vi "Frontend FPP v2.0.vi"() -> ()   [LabVIEW 2016]
panel:
  in  "Gate 2":T1={"Gate Start"=0.0, "Gate Stop"=2.0, "Gate Step (linear only)"=1.0, "Gate Compliance"=0.0001, "Gate PComp"=0.0, "Range mode"=0, "Range"=6} {"Range" max=11 scale=0.0..11.0; "Range mode" items=["Auto", "Limited", "Fixed"]; "Gate PComp" format="%^.2e"; "Gate Compliance" format="%^.2e"; "Gate Step (linear only)" format="%^.4e"; "Gate Stop" format="%^.4e"; "Gate Start" format="%^.4e"}
  in  "Drain":T2={"Drain Start"=0.0, "Drain Stop"=2.0, "Drain Compliance"=0.0001, "Drain Step"=1.0, "Drain PComp"=0.0, "Range mode"=0, "Range"=6} {"Range" max=11 scale=0.0..11.0; "Range mode" items=["Auto", "Limited", "Fixed"]; "Drain PComp" format="%^.2e"; "Drain Step" format="%^.4e"; "Drain Compliance" format="%^.2e"; "Drain Stop" format="%^.4e"; "Drain Start" format="%^.4e"}
  in  "Gate":T3={"Gate Start"=0.0, "Gate Stop"=2.0, "Gate Step"=1.0, "Gate Compliance"=0.0001, "Gate PComp"=0.0, "Range mode"=0, "Range"=6} {"Range" max=11 scale=0.0..11.0; "Range mode" items=["Auto", "Limited", "Fixed"]; "Gate PComp" format="%^.2e"; "Gate Compliance" format="%^.2e"; "Gate Step" format="%^.4e"; "Gate Stop" format="%^.4e"; "Gate Start" format="%^.4e"}
  in  "Drain 2":T4={"Drain Start"=0.0, "Drain Stop"=2.0, "Drain Compliance"=0.0001, "Drain Step (linear only)"=1.0, "Drain PComp"=0.0, "Range mode"=0, "Range"=6} {"Range" max=11 scale=0.0..11.0; "Range mode" items=["Auto", "Limited", "Fixed"]; "Drain PComp" format="%^.2e"; "Drain Step (linear only)" format="%^.4e"; "Drain Compliance" format="%^.2e"; "Drain Stop" format="%^.4e"; "Drain Start" format="%^.4e"}
  in  "Timings":T5={"integration time"=0, "Short/Long integration time"=0.00064, "hold time (sec)"=0.0, "delay time (sec)"=0.0, "Step Time (0 disables)"=0.0, "sweep method"=0, "Pulse period"=0.005, "Base voltage"=0.0, "Pulse width"=0.0005} {"Pulse width" min=0.0005 max=0.1 step=0.0001 format="%.4f"; "Base voltage" format="%^.4e"; "Pulse period" min=0.005 max=1.0 step=0.0001 format="%.4f"; "sweep method" items=["Continuous", "Pulsed"]; "Step Time (0 disables)" format="%.2f"; "delay time (sec)" format="%.4f"; "hold time (sec)" format="%.4f"; "Short/Long integration time" format="%^.0e"; "integration time" scale=0.0..2.0}
  in  "Panel controls":T6={"Emergency Stop"=refnum, "OutputGraph Max"=1e-05, "Text/Graph (text=false)"=FALSE} {"OutputGraph Max" format="%.2e"}
  in  "Panel Controls":T7={"Emergency Stop"=refnum, "TransGraph Max"=1e-05, "Text/Graph (text=false)"=FALSE} {"TransGraph Max" format="%.2e"}
  in  "Tab Control":enum32{"Characteristics", "Other parameters"}(tab)
  out "XY Graph 2":cluster{"Y data in":dbl[], "X data in":dbl[]}[](graph)
  in  "Integration time (long)":dbl=0.32 min=0.04 max=2.0 step=0.02 format="%.2f"
  in  "Integration time (short)":dbl=0.00064 min=8e-05 max=0.00192 step=8e-05 format="%^.0e"
  in  "Drain Range":u8(slide)=6 max=11 scale=0.0..11.0
  in  "Drain Range mode":u16(ring) items=["Auto", "Limited", "Fixed"]
  in  "Gate Range":u8(slide)=6 max=11 scale=0.0..11.0
  in  "Gate Range mode":u16(ring) items=["Auto", "Limited", "Fixed"]
  in  "Sampling mode":u32(slide) scale=0.0..4.0
  in  "Number of Samples":i32=500 min=0 step=1
  in  "Time":dbl=240.0 min=0.0 format="%.2f"
  in  "Drain":dbl=-10.0 min=-100.0 max=100.0 format="%.2f"
  in  "Gate":dbl=-60.0 min=-100.0 max=100.0 format="%.2f"
  in  "sweep method":u16(ring) items=["Continuous", "Pulsed"]
  out "Id":dbl format="%.2e"
  out "Ig":dbl format="%.2e"
  in  "Sweep Start":bool caption="Sweep start"
  in  "Interrupt run":bool
  in  "Running":bool=TRUE
  out "Path":path
  in  "integration time":u32(slide)=1 max=2 step=1 scale=0.0..2.0
  in  "sweep mode":u16(ring)=1 items=["Single", "Double"]
  in  "Transfer Start":bool
  in  "Output Start":bool
  in  "Drain: Step":dbl=-1.0 min=-100.0 max=100.0 format="%.2f"
  in  "Drain: Stop":dbl=-60.0 min=-100.0 max=100.0 format="%.2f"
  in  "Drain:Start":dbl min=-100.0 max=100.0 format="%.2f"
  in  "Gate: Step":dbl=-20.0 min=-100.0 max=100.0 format="%.2f"
  in  "Gate: Stop":dbl=-60.0 min=-100.0 max=100.0 format="%.2f"
  in  "Gate: Start":dbl min=-100.0 max=100.0 format="%.2f"
  out "XY Graph":cluster{"Y data in":dbl[], "X data in":dbl[]}[](graph)
  in  "Drain: Compliance":dbl=0.001 min=1e-12 max=0.02 format="%.8f"
  in  "Gate: Compliance":dbl=0.001 min=1e-12 max=0.02 format="%.8f"
  in  "Drain: Step":dbl=-5.0 min=-100.0 max=100.0 format="%.2f"
  in  "Drain: Stop":dbl=-10.0 min=-100.0 max=100.0 format="%.2f"
  in  "Drain:Start":dbl=-5.0 min=-100.0 max=100.0 format="%.2f"
  in  "Gate: Step":dbl=-1.0 min=-100.0 max=100.0 format="%.2f"
  in  "Gate: Stop":dbl=-60.0 min=-100.0 max=100.0 format="%.2f"
  in  "Gate: Start":dbl=10.0 min=-100.0 max=100.0 format="%.2f"
  in  "FPP - Source":u32(ring) items=["VSU1  ", "VSU2  "]
  in  "FPP - Drain":u32(ring)=1 items=["SMU1  ", "SMU2  ", "SMU3  ", "SMU4  ", "SMU5  ", "SMU6  "]
  in  "FPP - Gate":u32(ring)=2 items=["SMU1  ", "SMU2  ", "SMU3  ", "SMU4  ", "SMU5  ", "SMU6  "]
  in  "FPP - Probe 1":u32(ring) items=["SMU1  ", "SMU2  ", "SMU3  ", "SMU4  ", "SMU5  ", "SMU6  "]
  in  "FPP - Probe 2":u32(ring)=3 items=["SMU1  ", "SMU2  ", "SMU3  ", "SMU4  ", "SMU5  ", "SMU6  "]
  in  "Pulse width":dbl=0.0005 min=0.0005 max=0.1 step=0.0001 format="%.4f"
  in  "Base voltage":dbl min=-100.0 max=100.0 format="%.2f"
  in  "Pulse period":dbl=0.005 min=0.005 max=1.0 step=0.0001 format="%.4f"
  in  "Drain Power Compliance":dbl min=0.0 max=1.0 format="%.2f"
  in  "Gate Power\nCompliance":dbl min=0.0 max=1.0 format="%.2f"
  in  "OutputGraph Max":dbl=1e-05 format="%.2e"
  in  "TransGraph Max":dbl=1e-05 format="%.2e"
  in  "SPA Display":bool
  in  "Step delay /s":dbl min=0.0 max=1.0 format="%.2f"
  in  "hold time /s":dbl min=0.0 max=655.35 step=0.01 format="%.2f"
  in  "delay time /s":dbl min=0.0 max=65.535 step=0.0001 format="%.2f"
  in  "Decimal places in header":i8=1
  out "error out":errorcluster
  in  "VISA resource name in":refnum<visa-resource-name>="GPIB0::14::INSTR"
  # "Transfer Characteristics"
  # "Stress Measurements"
  # "V"
  # "V"
  # "V"
  # "Gate"
  # "V"
  # "V"
  # "V"
  # "V"
  # "Drain"
  # "V"
  # "s"
  # "Output Characteristics"
  # "V"
  # "V"
  # "V"
  # "Gate"
  # "V"
  # "V"
  # "Drain"
  # "V"
  # "For Four Point Probe measurements ONLY!"
  # "Vp1"
  # "Vp2"
  # "A"
  # "A"
  # "Pulsed mode settings"
  # "NOTE - THIS OVERRIDES THE COMPLIANCE VALUES!"
  # "A"
  # "A"
  # "Enter max power in Watts (max 1W)"
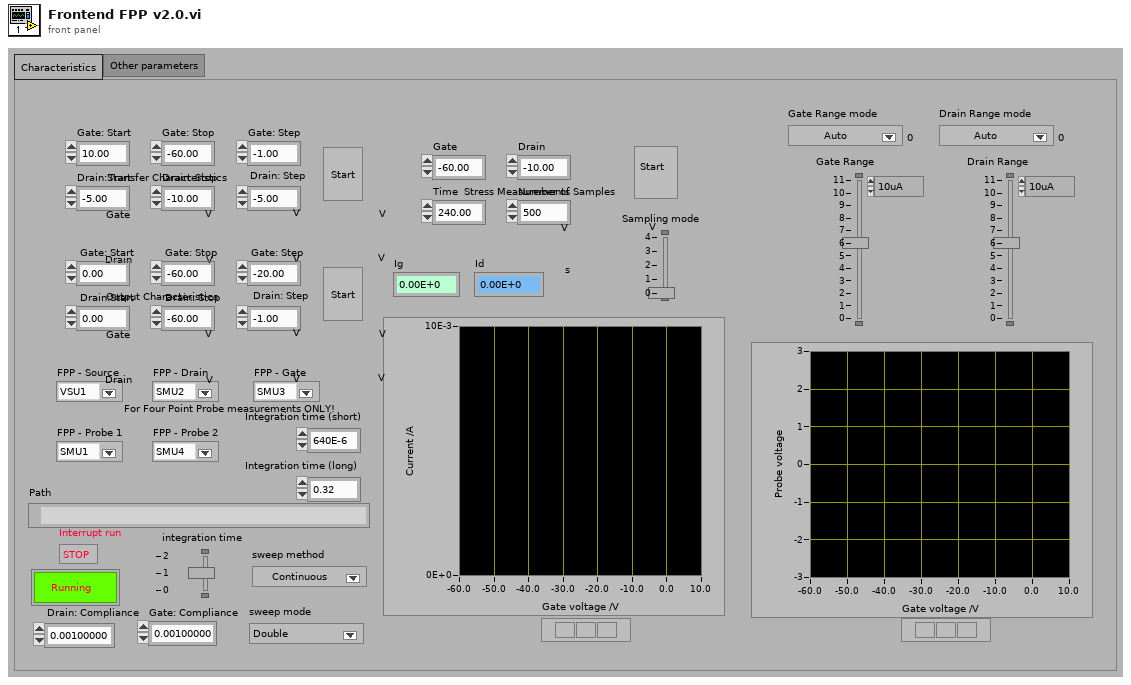
[diagram p1: front panel]
types:
  T1 = cluster{"Gate Start":dbl, "Gate Stop":dbl, "Gate Step (linear only)":dbl, "Gate Compliance":dbl, "Gate PComp":dbl, "Range mode":u16, "Range":u8}
  T2 = cluster{"Drain Start":dbl, "Drain Stop":dbl, "Drain Compliance":dbl, "Drain Step":dbl, "Drain PComp":dbl, "Range mode":u16, "Range":u8}
  T3 = cluster{"Gate Start":dbl, "Gate Stop":dbl, "Gate Step":dbl, "Gate Compliance":dbl, "Gate PComp":dbl, "Range mode":u16, "Range":u8}
  T4 = cluster{"Drain Start":dbl, "Drain Stop":dbl, "Drain Compliance":dbl, "Drain Step (linear only)":dbl, "Drain PComp":dbl, "Range mode":u16, "Range":u8}
  T5 = cluster{"integration time":u32, "Short/Long integration time":dbl, "hold time (sec)":dbl, "delay time (sec)":dbl, "Step Time (0 disables)":dbl, "sweep method":u16, "Pulse period":dbl, "Base voltage":dbl, "Pulse width":dbl}
  T6 = cluster{"Emergency Stop":refnum<vi>, "OutputGraph Max":dbl, "Text/Graph (text=false)":bool}
  T7 = cluster{"Emergency Stop":refnum<vi>, "TransGraph Max":dbl, "Text/Graph (text=false)":bool}
  T8 = cluster{"V2 Start":dbl, "V2 Step":dbl, "Number of points":i32}
  T9 = enum16{"open", "replace", "create", "open or create", "replace or create", "replace or create with confirmation"}
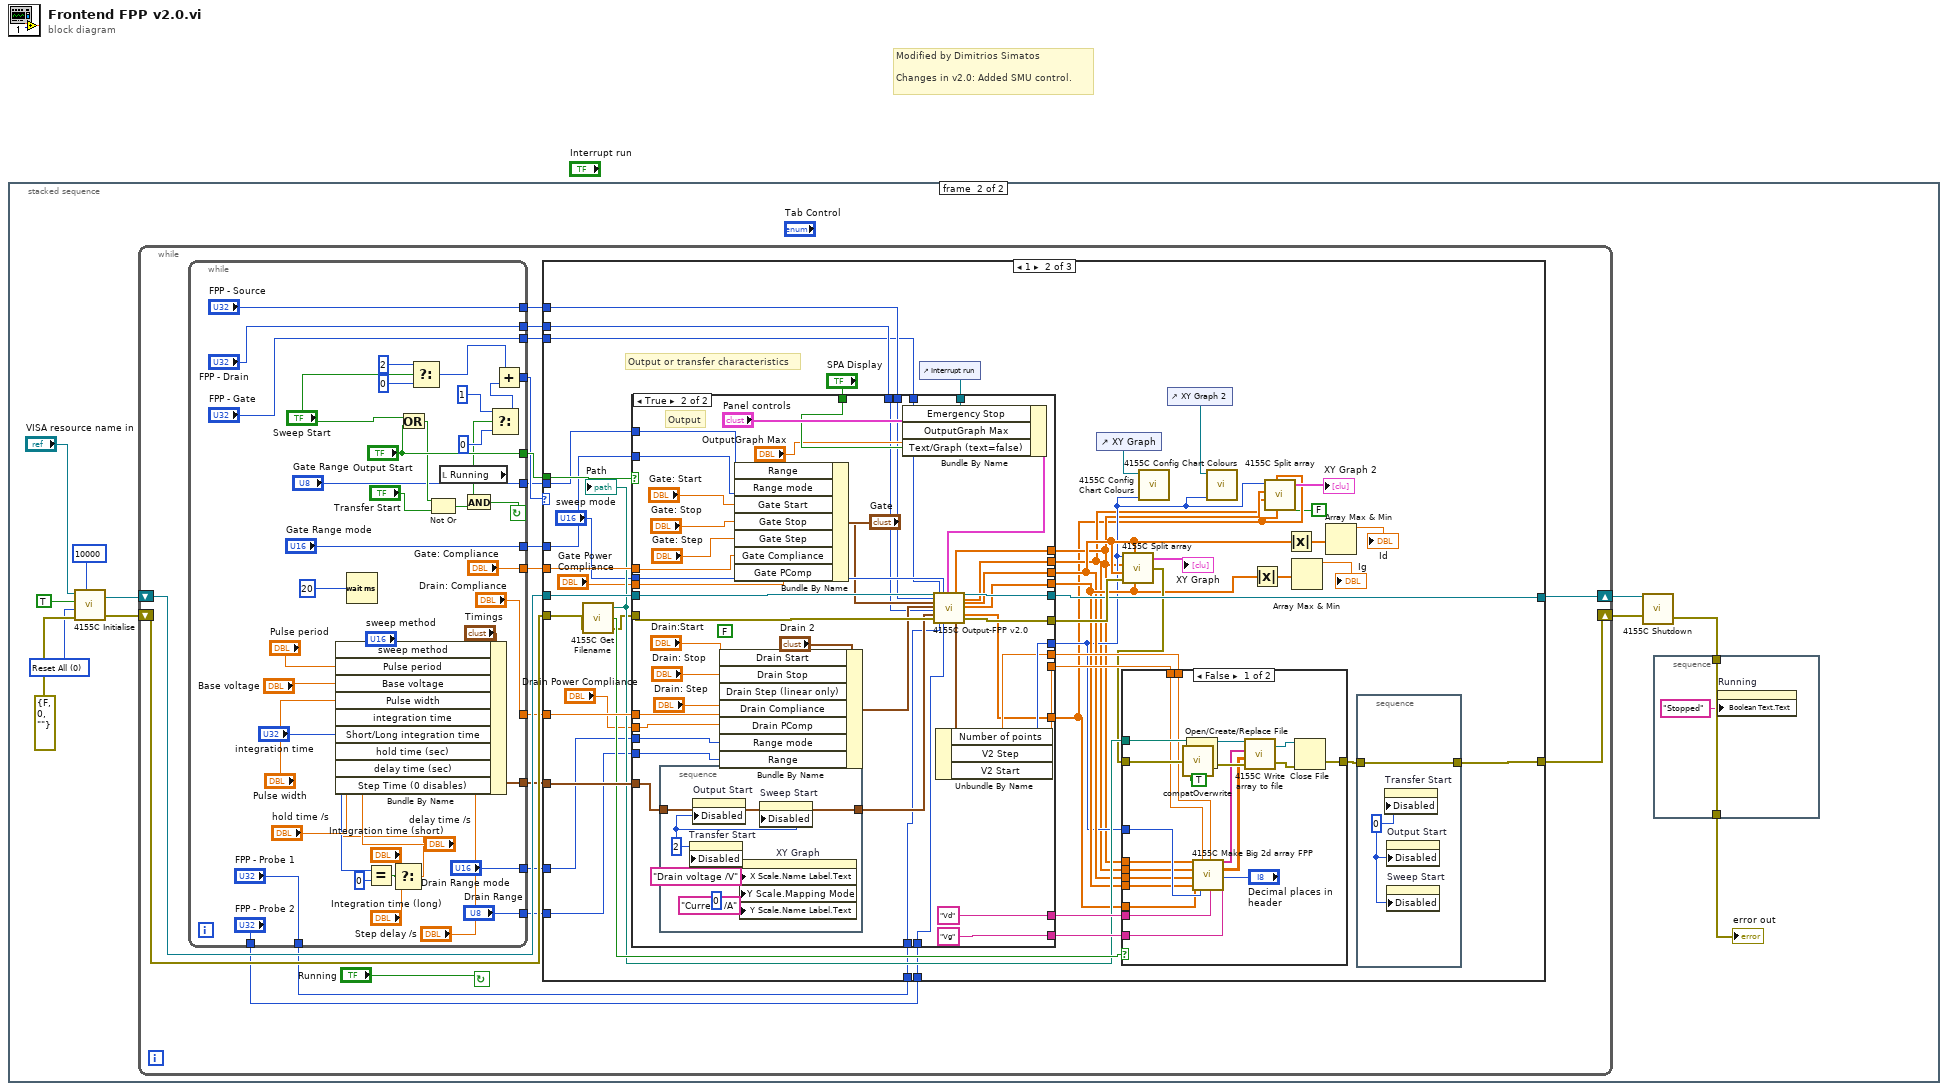
[diagram p0: block diagram]
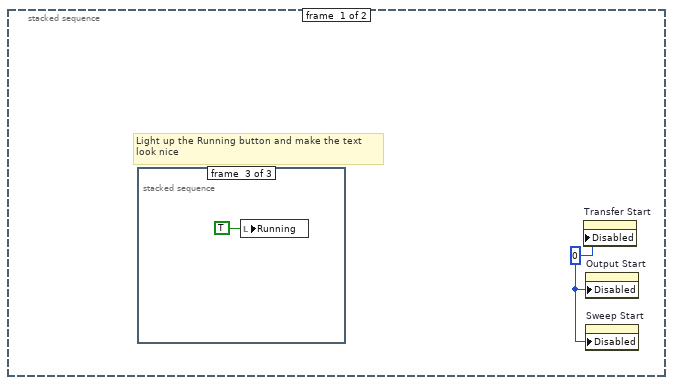
[diagram p2: hidden frame]
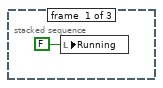
[diagram p3: hidden frame]
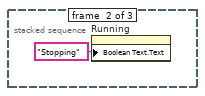
[diagram p4: hidden frame]
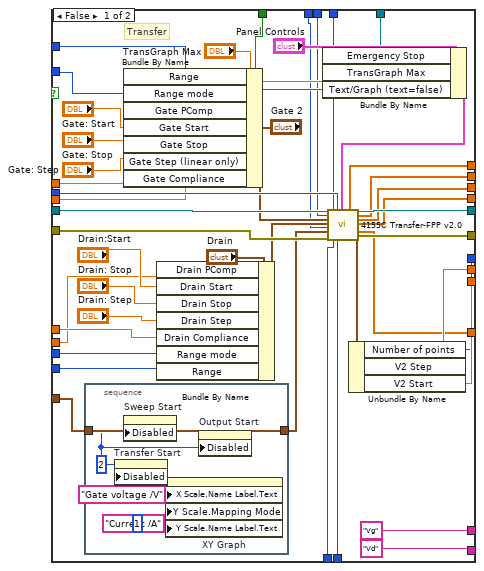
[diagram p7: hidden frame]
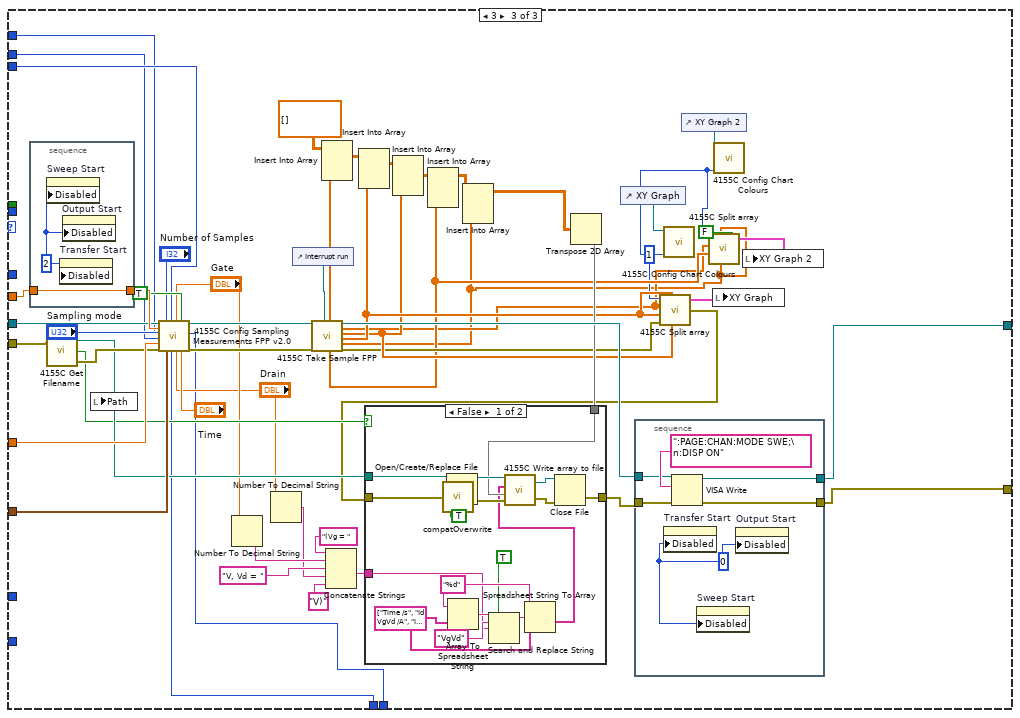
[diagram p8: hidden frame]
diagram:
  # "Modified by Dimitrios Simatos\n\nChanges in v2.0: Added SMU control."
  n1 = stacked-sequence {
    frame #0 {
      w1 = u8 0 ("Disabled")
      # "Light up the Running button and make the text\nlook nice"
      n2 = stacked-sequence {
        frame #0 {
          n3 = local write "Running"(FALSE ("Running")) -> ()
        }
        frame #1 {
          n4 = property on="Running" class="Bool (strict)"("Boolean Text.Text"="Stopping") -> ()  [unwired: 2 in, 2 out]
        }
        frame #2 {
          (unwired) FALSE ("Running")
          n5 = local write "Running"(TRUE ("Running")) -> ()
        }
      }
      n6 = property on="Transfer Start" class="Bool (strict)"("Disabled"=w1) -> ()  [unwired: 2 in, 2 out]
      n7 = property on="Output Start" class="Bool (strict)"("Disabled"=w1) -> ()  [unwired: 2 in, 2 out]
      n8 = property on="Sweep Start" class="Bool (strict)"("Disabled"=w1) -> ()  [unwired: 2 in, 2 out]
    }
    frame #1 {
      w11 = u16 0 items=["Reset All", "Partial reset"] ("Type of reset")
      n9 = call "4155C Initialise.vi"("VISA resource name in"="VISA resource name in", "Reset"=TRUE, "Type of reset"=w11, "error in (no error)"=errorcluster {"status"=FALSE, "code"=0, "source"=""}, "VISA Timeout Value"=u32 10000) -> ("VISA Resource Name out"=w10:refnum<visa-resource-name>, "error out"=w9:errorcluster)
      n10 = while {
        shift-left: w10 -> [w29]
        shift-right: [w31] -> w5
        shift-left: w9 -> [w30]
        shift-right: [w32] -> w6
        stop <- "Running" continue-if-true
        n11 = while {
          tunnel: ["Gate Range"] -> w21
          tunnel: ["Gate Range mode"] -> w22
          tunnel: ["Drain Range"] -> w23
          tunnel: ["Drain Range mode"] -> w24
          tunnel: ["Drain: Compliance"] -> w25
          tunnel: [w59] -> w26
          tunnel: ["Gate: Compliance"] -> w27
          tunnel: [w65] -> w28
          tunnel: ["Output Start"] -> w33
          tunnel: ["FPP - Source"] -> w20
          tunnel: ["FPP - Drain"] -> w19
          tunnel: ["FPP - Gate"] -> w18
          tunnel: ["FPP - Probe 2"] -> w17
          tunnel: ["FPP - Probe 1"] -> w16
          stop <- w74 continue-if-true
          n12 = Wait (ms)(milliseconds to wait=u32 20) -> ()  [unwired: 1 out]
          n13 = Equal?(x="integration time", y=u32 0) -> (x = y?=w56:bool)
          n14 = Select(t="Integration time (short)", s=w56, f="Integration time (long)") -> (s? t:f=w53:dbl)
          n15 = Bundle By Name(cluster="Timings", "sweep method"="sweep method", "Pulse period"="Pulse period", "Base voltage"="Base voltage", "Pulse width"="Pulse width", "integration time"="integration time", "Short/Long integration time"=w53, "hold time (sec)"="hold time /s", "delay time (sec)"="delay time /s", "Step Time (0 disables)"="Step delay /s") -> (w59:T5)
          n16 = Or(x="Sweep Start", y="Output Start") -> (x .or. y?=w71:bool)
          n17 = Select(t=i8 2, s="Sweep Start", f=i8 0) -> (s? t:f=w41:i8)
          n18 = Not Or(1:"Transfer Start", 2:w71) -> (0:w73:bool)
          n19 = local read "Running"() -> (w68:bool)
          n20 = And(x=w68, y=w73) -> (x .and. y?=w74:bool)
          n21 = Select(t=i8 1, s=w68, f=i8 0) -> (s? t:f=w64:i8)
          n22 = Add(x=w41, y=w64) -> (x+y=w65:i8)
        }
        n23 = case shown="1" w28 {
          tunnel: w33 -> [_ w124 _]
          tunnel: w26 -> [_ w123 w296]
          tunnel: w27 -> [_ w122 w304]
          tunnel: w25 -> [_ w121 w300]
          tunnel: [w77 w112 w302] -> w32
          tunnel: [w76 w115 w303] -> w31
          tunnel: w30 -> [w77 w106 w291]
          tunnel: w29 -> [w76 w114 w290]
          tunnel: w24 -> [_ w96 _]
          tunnel: w23 -> [_ w95 _]
          tunnel: w22 -> [_ w94 _]
          tunnel: w21 -> [_ w93 _]
          tunnel: w20 -> [_ w82 w255]
          tunnel: w19 -> [_ w81 w254]
          tunnel: w18 -> [_ w80 w256]
          tunnel: w17 -> [_ w79 w253]
          tunnel: w16 -> [_ w78 w252]
          frame 0, Default {
            # "Someone's deselected the running button so just shutdown..."
          }
          frame 1 {
            # "Output or transfer characteristics"
            n24 = call "4155C Get Filename.vi"("error in (no error)"=w106) -> ("error out"=w105:errorcluster, "cancelled"=w111:bool, "path"=w110:path)  [unwired: 2 in]
            "Path" <- w110
            n25 = control-ref of="Interrupt run"() -> (w107:refnum<vi>)
            n26 = case shown="True" w124 {
              tunnel: w114 -> [w181 w232]
              tunnel: w105 -> [w180 w231]
              tunnel: w123 -> [w184 w237]
              tunnel: w122 -> [w190 w244]
              tunnel: w121 -> [w195 w243]
              tunnel: "sweep mode" -> [w189 w242]
              tunnel: [w157 w210] -> w86
              tunnel: [w156 w209] -> w85
              tunnel: [w159 w208] -> w92
              tunnel: [w158 w207] -> w97
              tunnel: [w188 w241] -> w115
              tunnel: [w187 w240] -> w120
              tunnel: [w160 w213] -> w87
              tunnel: [w161 w212] -> w118
              tunnel: [w162 w211] -> w119
              tunnel: ["Vg" "Vd"] -> w117
              tunnel: ["Vd" "Vg"] -> w116
              tunnel: w107 -> [w178 w230]
              tunnel: "SPA Display" -> [w177 w228]
              tunnel: "Drain Power Compliance" -> [w173 w225]
              tunnel: "Gate Power\nCompliance" -> [w174 w224]
              tunnel: w96 -> [w165 w218]
              tunnel: w95 -> [w164 w217]
              tunnel: w94 -> [w166 w216]
              tunnel: w93 -> [w167 w215]
              tunnel: [w155 w206] -> w84
              tunnel: w82 -> [w154 w204]
              tunnel: w81 -> [w153 w203]
              tunnel: w80 -> [w152 w205]
              tunnel: w79 -> [w151 w202]
              tunnel: w78 -> [w150 w201]
              frame False {
                # "Transfer"
                n27 = stacked-sequence {
                  tunnel: w184 -> [w199]
                  tunnel: [w199] -> w172
                  frame #0 {
                    w197 = u8 2 ("Disabled")
                    n28 = property on="Transfer Start" class="Bool (strict)"("Disabled"=w197) -> ()  [unwired: 2 in, 2 out]
                    n29 = property on="Sweep Start" class="Bool (strict)"("Disabled"=w197) -> ()  [unwired: 2 in, 2 out]
                    n30 = property on="XY Graph" class="XYGraph (strict)"("X Scale.Name Label.Text"="Gate voltage /V", "Y Scale.Mapping Mode"=u8 1, "Y Scale.Name Label.Text"="Current /A") -> ()  [unwired: 2 in, 2 out]
                    n31 = property on="Output Start" class="Bool (strict)"("Disabled"=w197) -> ()  [unwired: 2 in, 2 out]
                  }
                }
                n32 = Bundle By Name(cluster="Gate 2", "Range"=w167, "Range mode"=w166, "Gate PComp"=w174, "Gate Start"="Gate: Start", "Gate Stop"="Gate: Stop", "Gate Step (linear only)"="Gate: Step", "Gate Compliance"=w190) -> (w168:T1)
                n33 = Bundle By Name(cluster="Drain", "Drain PComp"=w173, "Drain Start"="Drain:Start", "Drain Stop"="Drain: Stop", "Drain Step"="Drain: Step", "Drain Compliance"=w195, "Range mode"=w165, "Range"=w164) -> (w170:T2)
                n34 = Bundle By Name(cluster="Panel Controls", "Emergency Stop"=w178, "TransGraph Max"="TransGraph Max", "Text/Graph (text=false)"=w177) -> (w175:T7)
                n35 = call "4155C Transfer-FPP v2.0.vi"("VISA resource name in"=w181, "FPP - Source"=w154, "Gate"=w168, "Drain"=w170, "FPP - Drain"=w153, "Timings"=w172, "error in (no error)"=w180, "FPP - Gate"=w152, "FPP - Probe 1"=w150, "sweep mode"=w189, "FPP - Probe 2"=w151, "Panel Controls"=w175) -> ("VG"=w157:dbl[], "Outparams"=w163:T8, "VISA Resource Name out"=w188:refnum<visa-resource-name>, "Vprobe2"=w156:dbl[], "ID"=w159:dbl[], "IG"=w158:dbl[], "Vprobe1"=w155:dbl[], "error out"=w187:errorcluster)  [unwired: 8 in]
                n36 = Unbundle By Name(w163) -> ("Number of points"=w160:i32, "V2 Step"=w161:dbl, "V2 Start"=w162:dbl)
              }
              frame True {
                (unwired) FALSE ("Logarithmic")
                # "Output"
                n37 = stacked-sequence {
                  tunnel: w237 -> [w250]
                  tunnel: [w250] -> w223
                  frame #0 {
                    w248 = u8 2 ("Disabled")
                    n38 = property on="Transfer Start" class="Bool (strict)"("Disabled"=w248) -> ()  [unwired: 2 in, 2 out]
                    n39 = property on="Output Start" class="Bool (strict)"("Disabled"=w248) -> ()  [unwired: 2 in, 2 out]
                    n40 = property on="XY Graph" class="XYGraph (strict)"("X Scale.Name Label.Text"="Drain voltage /V", "Y Scale.Mapping Mode"=u8 0, "Y Scale.Name Label.Text"="Current /A") -> ()  [unwired: 2 in, 2 out]
                    n41 = property on="Sweep Start" class="Bool (strict)"("Disabled"=w248) -> ()  [unwired: 2 in, 2 out]
                  }
                }
                n42 = Bundle By Name(cluster="Drain 2", "Drain Start"="Drain:Start", "Drain Stop"="Drain: Stop", "Drain Step (linear only)"="Drain: Step", "Drain Compliance"=w243, "Drain PComp"=w225, "Range mode"=w218, "Range"=w217) -> (w221:T4)
                n43 = Bundle By Name(cluster="Gate", "Range"=w215, "Range mode"=w216, "Gate Start"="Gate: Start", "Gate Stop"="Gate: Stop", "Gate Step"="Gate: Step", "Gate Compliance"=w244, "Gate PComp"=w224) -> (w219:T3)
                n44 = Bundle By Name(cluster="Panel controls", "Emergency Stop"=w230, "OutputGraph Max"="OutputGraph Max", "Text/Graph (text=false)"=w228) -> (w226:T6)
                n45 = call "4155C Output-FPP v2.0.vi"("VISA resource name in"=w232, "FPP - Source"=w204, "Gate"=w219, "Drain"=w221, "FPP - Drain"=w203, "Timings"=w223, "error in (no error)"=w231, "FPP - Gate"=w205, "FPP - Probe 1"=w201, "sweep mode"=w242, "FPP - Probe 2"=w202, "Panel controls"=w226) -> ("VD"=w210:dbl[], "Outparams"=w214:T8, "VISA Resource Name out"=w241:refnum<visa-resource-name>, "Vprobe2"=w209:dbl[], "ID"=w208:dbl[], "IG"=w207:dbl[], "Vprobe1"=w206:dbl[], "error out"=w240:errorcluster)  [unwired: 8 in]
                n46 = Unbundle By Name(w214) -> ("Number of points"=w213:i32, "V2 Step"=w212:dbl, "V2 Start"=w211:dbl)
              }
            }
            n47 = control-ref of="XY Graph"() -> (w108:refnum<vi>)
            n48 = call "4155C Split array.vi"("Number of VAR2 steps"=w87, "Y2 data in"=w92, "X data in"=w86, "Y1 data in"=w92, "Y3 data in"=w97, "error in (no error)"=w120) -> ("Array of clusters"=→"XY Graph":cluster{"Y data in":dbl[], "X data in":dbl[]}[], "error out"=w104:errorcluster)  [unwired: 1 in]
            n49 = case shown="False" w111 {
              tunnel: w104 -> [w147 w149]
              tunnel: [w142 w149] -> w113
              tunnel: w110 -> [w146 _]
              tunnel: w87 -> [w140 _]
              tunnel: w92 -> [w130 _]
              tunnel: w86 -> [w132 _]
              tunnel: w85 -> [w131 _]
              tunnel: w97 -> [w129 _]
              tunnel: w119 -> [w134 _]
              tunnel: w118 -> [w135 _]
              tunnel: w117 -> [w139 _]
              tunnel: w116 -> [w138 _]
              tunnel: w84 -> [w128 _]
              frame False {
                n50 = call <vilib>:"compatOverwrite.vi"("overwrite (F)"=TRUE) -> ("overwrite?"=w127:T9)
                n51 = Open/Create/Replace File(file path (use dialog)=w146, error in=w147, operation (0:open)=w127) -> (refnum out=w144:refnum<file>, error out=w145:errorcluster)  [unwired: 3 in, 1 out]
                n52 = call "4155C Make Big 2d array FPP.vi"("1D Var1"=w132, "1d ID"=w130, "1d Vp2"=w131, "1d IG"=w129, "1d Vp1"=w128, "VAR2 START"=w134, "Number of VAR2 steps"=w140, "VAR2 STEP"=w135, "VAR1 Name"=w139, "Decimal places in header"="Decimal places in header", "VAR2 Name"=w138) -> ("Header array"=w136:string[], "Data array"=w137:dbl[][])  [unwired: 15 in]
                n53 = call "4155C Write array to file.vi"("Byte Stream File Refnum"=w144, "Header"=w136, "Data Array"=w137, "error in (no error)"=w145) -> ("dup refnum"=w141:refnum<file>, "error out"=w143:errorcluster)  [unwired: 1 in]
                n54 = Close File(refnum=w141, error in=w143) -> (error out=w142:errorcluster)  [unwired: 1 out]
              }
              frame True {
              }
            }
            n55 = call "4155C Config Chart Colours.vi"("Numeric"=w87, "XY Graph 2"=w108) -> ()  [unwired: 6 in]
            n56 = control-ref of="XY Graph 2"() -> (w89:refnum<vi>)
            n57 = call "4155C Config Chart Colours.vi"("Numeric"=w87, "XY Graph 2"=w89) -> ()  [unwired: 6 in]
            n58 = Absolute Value(x=w97) -> (abs(x)=w99:dbl[])
            n59 = call "4155C Split array.vi"("Number of VAR2 steps"=w87, "Y2 data in"=w84, "X data in"=w86, "Y1 data in"=w85, "Y3 data in"=w84, "Absolute val?"=FALSE) -> ("Array of clusters"=→"XY Graph 2":cluster{"Y data in":dbl[], "X data in":dbl[]}[])  [unwired: 1 in, 1 out]
            n60 = Absolute Value(x=w92) -> (abs(x)=w98:dbl[])
            n61 = Array Max & Min(array=w99) -> (max value=→"Ig":dbl)  [unwired: 3 out]
            n62 = Array Max & Min(array=w98) -> (max value=→"Id":dbl)  [unwired: 3 out]
            n63 = stacked-sequence {
              tunnel: w113 -> [w126]
              tunnel: [w126] -> w112
              frame #0 {
                w125 = u8 0 ("Disabled")
                n64 = property on="Transfer Start" class="Bool (strict)"("Disabled"=w125) -> ()  [unwired: 2 in, 2 out]
                n65 = property on="Output Start" class="Bool (strict)"("Disabled"=w125) -> ()  [unwired: 2 in, 2 out]
                n66 = property on="Sweep Start" class="Bool (strict)"("Disabled"=w125) -> ()  [unwired: 2 in, 2 out]
              }
            }
          }
          frame 3 {
            w260 = 1 ("Numeric")
            n67 = stacked-sequence {
              tunnel: w304 -> [w331]
              tunnel: [w331] -> w301
              frame #0 {
                w330 = u8 2 ("Disabled")
                n68 = property on="Sweep Start" class="Bool (strict)"("Disabled"=w330) -> ()  [unwired: 2 in, 2 out]
                n69 = property on="Transfer Start" class="Bool (strict)"("Disabled"=w330) -> ()  [unwired: 2 in, 2 out]
                n70 = property on="Output Start" class="Bool (strict)"("Disabled"=w330) -> ()  [unwired: 2 in, 2 out]
              }
            }
            n71 = call "4155C Get Filename.vi"("error in (no error)"=w291) -> ("error out"=w289:errorcluster, "cancelled"=w280:bool, "path"=w281:path)  [unwired: 2 in]
            n72 = local write "Path"(w281) -> ()
            n73 = call "4155C Config Sampling Measurements FPP v2.0.vi"("VISA session"=w290, "Gate Compliance"=w301, "FPP - Source"=w255, "FPP - Drain"=w254, "Drain Compliance"=w300, "error in (no error)"=w289, "Num Points"="Number of Samples", "Timings"=w296, "FPP - Gate"=w256, "FPP - Probe 1"=w252, "Vg"="Gate", "Vd"="Drain", "Display on/off"=TRUE, "Sample time"="Time", "Sampling mode"="Sampling mode", "FPP - Probe 2"=w253) -> ("dup VISA resource name"=w297:refnum<visa-resource-name>, "error out"=w298:errorcluster)  [unwired: 2 in]
            n74 = Number To Decimal String(number="Gate") -> (decimal integer string=w278:string)  [unwired: 1 in]
            n75 = Number To Decimal String(number="Drain") -> (decimal integer string=w276:string)  [unwired: 1 in]
            n76 = control-ref of="Interrupt run"() -> (w292:refnum<vi>)
            n77 = call "4155C Take Sample FPP.vi"("VISA resource name in"=w297, "error in (no error)"=w298, "Emergency Stop"=w292) -> ("Time"=w258:dbl[], "Vp1"=w262:dbl[], "VISA Resource Name out"=w299:refnum<visa-resource-name>, "Ig"=w270:dbl[], "Id"=w271:dbl[], "Vp2"=w257:dbl[], "error out"=w269:errorcluster)  [unwired: 10 in]
            n78 = Insert Into Array(array=dbl[][] [] ("Input Array"), new element=w258) -> (w288:dbl[][])  [unwired: 2 in]
            n79 = Concatenate Strings("(Vg = " ("Substring"), w278, "V, Vd = " ("Substring"), w276, "V)" ("Substring")) -> (w274:string)
            n80 = Insert Into Array(array=w288, new element=w271) -> (w287:dbl[][])  [unwired: 2 in]
            n81 = Insert Into Array(array=w287, new element=w270) -> (w286:dbl[][])  [unwired: 2 in]
            n82 = Insert Into Array(array=w286, new element=w262) -> (w284:dbl[][])  [unwired: 2 in]
            n83 = Insert Into Array(array=w284, new element=w257) -> (w264:dbl[][])  [unwired: 2 in]
            n84 = Transpose 2D Array(2D array=w264) -> (transposed array=w282:dbl[][])
            n85 = control-ref of="XY Graph"() -> (w273:refnum<vi>)
            n86 = call "4155C Split array.vi"("Number of VAR2 steps"=w260, "Y2 data in"=w271, "X data in"=w258, "Y1 data in"=w271, "Y3 data in"=w270, "error in (no error)"=w269) -> ("Array of clusters"=w272:cluster{"Y data in":dbl[], "X data in":dbl[]}[], "error out"=w268:errorcluster)  [unwired: 1 in]
            n87 = case shown="False" w280 {
              tunnel: w268 -> [w321 w323]
              tunnel: [w316 w323] -> w283
              tunnel: w281 -> [w320 _]
              tunnel: w282 -> [w314 _]
              tunnel: w274 -> [w306 _]
              frame False {
                w307 = string[] ["Time /s", "Id VgVd /A", "Ig VgVd /A", "Vp1 VgVd /V", "Vp2 VgVd /V"] ("Header")
                w311 = "%d" ("format string")
                n88 = call <vilib>:"compatOverwrite.vi"("overwrite (F)"=TRUE) -> ("overwrite?"=w305:T9)
                n89 = Open/Create/Replace File(file path (use dialog)=w320, error in=w321, operation (0:open)=w305) -> (refnum out=w318:refnum<file>, error out=w319:errorcluster)  [unwired: 3 in, 1 out]
                n90 = Array To Spreadsheet String(array=w307, 3:w311) -> (spreadsheet string=w313:string)  [unwired: 1 in]
                n91 = Search and Replace String(replace all?=TRUE ("replace all? (F)"), input string=w313, search string="VgVd", replace string=w306) -> (result string=w309:string)  [unwired: 4 in, 3 out]
                n92 = Spreadsheet String To Array(format string=w311, spreadsheet string=w309, array type (2D Dbl)=w307) -> (array=w308:string[])  [unwired: 1 in]
                n93 = call "4155C Write array to file.vi"("Byte Stream File Refnum"=w318, "Header"=w308, "Data Array"=w314, "error in (no error)"=w319) -> ("dup refnum"=w315:refnum<file>, "error out"=w317:errorcluster)  [unwired: 1 in]
                n94 = Close File(refnum=w315, error in=w317) -> (error out=w316:errorcluster)  [unwired: 1 out]
              }
              frame True {
              }
            }
            n95 = stacked-sequence {
              tunnel: [w326] -> w303
              tunnel: [w325] -> w302
              tunnel: w299 -> [w328]
              tunnel: w283 -> [w327]
              frame #0 {
                w324 = u8 0 ("Disabled")
                n96 = property on="Transfer Start" class="Bool (strict)"("Disabled"=w324) -> ()  [unwired: 2 in, 2 out]
                n97 = VISA Write(VISA resource name=w328, write buffer=":PAGE:CHAN:MODE SWE;\n:DISP ON" ("write buffer (\"\")"), error in (no error)=w327) -> (VISA resource name out=w326:refnum<visa-resource-name>, error out=w325:errorcluster)  [unwired: 1 out]
                n98 = property on="Sweep Start" class="Bool (strict)"("Disabled"=w324) -> ()  [unwired: 2 in, 2 out]
                n99 = property on="Output Start" class="Bool (strict)"("Disabled"=w324) -> ()  [unwired: 2 in, 2 out]
              }
            }
            n100 = call "4155C Config Chart Colours.vi"("Numeric"=w260, "XY Graph 2"=w273) -> ()  [unwired: 6 in]
            n101 = control-ref of="XY Graph 2"() -> (w263:refnum<vi>)
            n102 = call "4155C Split array.vi"("Number of VAR2 steps"=w260, "Y2 data in"=w257, "X data in"=w258, "Y1 data in"=w262, "Y3 data in"=w257, "Absolute val?"=FALSE) -> ("Array of clusters"=w261:cluster{"Y data in":dbl[], "X data in":dbl[]}[])  [unwired: 1 in, 1 out]
            n103 = local write "XY Graph"(w272) -> ()
            n104 = call "4155C Config Chart Colours.vi"("Numeric"=w260, "XY Graph 2"=w263) -> ()  [unwired: 6 in]
            n105 = local write "XY Graph 2"(w261) -> ()
          }
        }
      }
      n106 = call "4155C Shutdown.vi"("VISA resource name in"=w5, "error in (no error)"=w6) -> ("error out"=w8:errorcluster)  [unwired: 4 in]
      n107 = stacked-sequence {
        tunnel: w8 -> [w333]
        tunnel: [w333] -> w7
        frame #0 {
          n108 = property on="Running" class="Bool (strict)"("Boolean Text.Text"="Stopped") -> ()  [unwired: 2 in, 2 out]
        }
      }
      "error out" <- w7
    }
  }
